vi "ConfigurePigeonMP.vi"(8 "Pigeon Talon":T1, 9 "Pigeon":T6 {"Type" items=["CAN"=352321536, "TalonSRX"=33554432]}, 10 "Right Side":T1, 11 "Left Side":T1) -> (1 "Pigeon":T6 {"Type" items=["CAN"=352321536, "TalonSRX"=33554432]}, 2 "Right Side":T1, 3 "Left Side":T1)   [LabVIEW 2018]
uses:
  <vilib>/Rock Robotics/WPI/ThirdParty/Phoenix-LabVIEW/Pigeon IMU/CTRE_PigeonIMU_DeviceRef.ctl
  <vilib>/Rock Robotics/WPI/ThirdParty/Phoenix-LabVIEW/Pigeon IMU/CTRE_PigeonIMU_ConnectionType.ctl
  <vilib>/Rock Robotics/WPI/MotorControl/WPI_MotorControlDeviceRef.ctl
  <vilib>/Rock Robotics/WPI/MotorControl/WPI_MotorControlType.ctl
  <vilib>/Rock Robotics/SystemInterfaces/DIO/FPGA_DIOPWMChannel.ctl
  <vilib>/Rock Robotics/WPI/PWM/WPI_PWMDeadband.ctl
  <vilib>/Rock Robotics/SystemInterfaces/DIO/FPGA_DIOChannel.ctl
  <vilib>/Rock Robotics/WPI/ThirdParty/Phoenix-LabVIEW/Motor Controller/Controls/CTRE_Phoenix_MotorControl_FeedbackDevice.ctl
  <vilib>/Rock Robotics/WPI/ThirdParty/Phoenix-LabVIEW/Motor Controller/Controls/CTRE_Phoenix_MotorControl_RemoteSourceType.ctl
  <vilib>/Rock Robotics/WPI/ThirdParty/Phoenix-LabVIEW/Motor Controller/Controls/CTRE_Phoenix_MotorControl_SensorTermFeedbackDevice_Enhanced.ctl
  <vilib>/Rock Robotics/WPI/ThirdParty/Phoenix-LabVIEW/Motor Controller/Controls/CTRE_Phoenix_MotorControl_StatusFrameEnhanced.ctl
  <vilib>/Rock Robotics/WPI/ThirdParty/Phoenix-LabVIEW/Motor Controller/Controls/CTRE_Phoenix_MotorControl_NeutralMode.ctl
  <vilib>/Rock Robotics/WPI/ThirdParty/Phoenix-LabVIEW/Motor Controller/Controls/CTRE_Phoenix_MotorControl_ControlMode.ctl
  <vilib>/Rock Robotics/WPI/ThirdParty/Phoenix-LabVIEW/Controls/CTRE_Phoenix_Params.ctl
  <vilib>/Rock Robotics/WPI/ThirdParty/Phoenix-LabVIEW/Motor Controller/Controls/CTRE_Phoenix_MotorControl_ControlFrameEnhanced.ctl
  Constants.vi
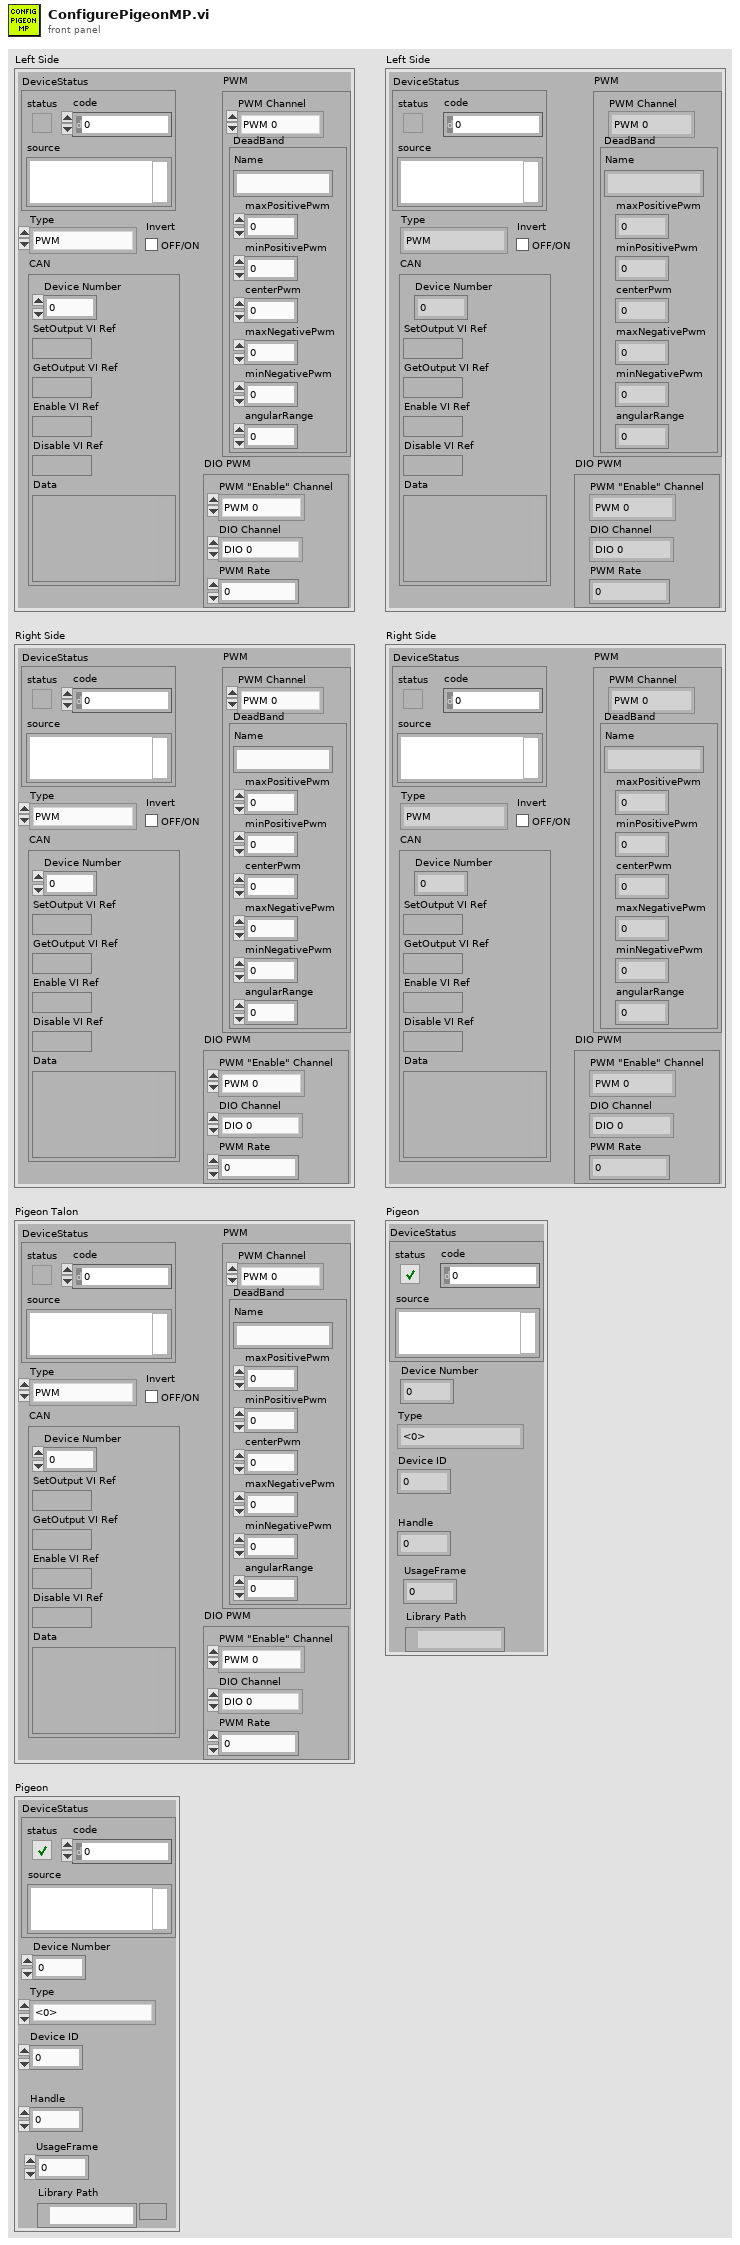
[diagram p1: front panel]
types:
  T1 = typedef "WPI_MotorControlDeviceRef.ctl" = cluster{"DeviceStatus":errorcluster, "Type":T2, "PWM":cluster{"PWM Channel":T3, "DeadBand":T4}, "CAN":cluster{"Device Number":u8, "SetOutput VI Ref":variant, "GetOutput VI Ref":variant, "Enable VI Ref":variant, "Disable VI Ref":variant, "Data":variant}, "Invert":bool, "DIO PWM":cluster{"PWM \"Enable\" Channel":T3, "DIOChannel":T5, "PWM Rate":dbl}}
  T2 = typedef "WPI_MotorControlType.ctl" = enum16{"PWM", "CAN", "DIO PWM"}
  T3 = typedef "FPGA_DIOPWMChannel.ctl" = enum8{"PWM 0", "PWM 1", "PWM 2", "PWM 3", "PWM 4", "PWM 5", "PWM 6", "PWM 7", "PWM 8", "PWM 9", "PWM MXP 0", "PWM MXP 1", "PWM MXP 2", "PWM MXP 3", "PWM MXP 4", "PWM MXP 5", "PWM MXP 6", "PWM MXP 7", "PWM MXP 8", "PWM MXP 9", "Invalid"}
  T4 = typedef "WPI_PWMDeadband.ctl" = cluster{"Name":string, "maxPositivePwm":i32, "minPositivePwm":i32, "centerPwm":i32, "maxNegativePwm":i32, "minNegativePwm":i32, "angularRange":u16}
  T5 = typedef "FPGA_DIOChannel.ctl" = enum8{"DIO 0", "DIO 1", "DIO 2", "DIO 3", "DIO 4", "DIO 5", "DIO 6", "DIO 7", "DIO 8", "DIO 9", "DIO MXP 0", "DIO MXP 1", "DIO MXP 2", "DIO MXP 3", "DIO MXP 4", "DIO MXP 5", "DIO MXP 6", "DIO MXP 7", "DIO MXP 8", "DIO MXP 9", "DIO MXP 10", "DIO MXP 11", "DIO MXP 12", "DIO MXP 13", "DIO MXP 14", "DIO MXP 15", "SPI Port CS1", "SPI Port CS2", "SPI Port CS3", "SPI Port MISO", "SPI Port MOSI", "Invalid"}
  T6 = typedef "CTRE_PigeonIMU_DeviceRef.ctl" = cluster{"DeviceStatus":errorcluster, "Device Number":u8, "Type":T7, "Device ID":u32, "Handle":u64, "UsageFrame":u32, "Library Path":path}
  T7 = typedef "CTRE_PigeonIMU_ConnectionType.ctl" = u32
  T8 = typedef "CTRE_Phoenix_MotorControl_ControlFrameEnhanced.ctl" = u32
  T9 = typedef "CTRE_Phoenix_MotorControl_StatusFrameEnhanced.ctl" = u16
  T10 = typedef "CTRE_Phoenix_Params.ctl" = u16
  T11 = typedef "CTRE_Phoenix_MotorControl_ControlMode.ctl" = u16
  T12 = typedef "CTRE_Phoenix_MotorControl_NeutralMode.ctl" = enum8{"EEPROMSetting", "Override to Coast", "Override to Brake"}
  T13 = typedef "CTRE_Phoenix_MotorControl_FeedbackDevice.ctl" = i8
  T14 = typedef "CTRE_Phoenix_MotorControl_SensorTermFeedbackDevice_Enhanced.ctl" = i8
  T15 = typedef "CTRE_Phoenix_MotorControl_RemoteSourceType.ctl" = enum16{"Off", "Talon SRX Selected Sensor", "Pigeon IMU Yaw", "Pigeon IMU Pitch", "Pigeon IMU Roll", "CANifier Quadrature", "CANifier PWM Input 0", "CANifier PWM Input 1", "CANifier PWM Input 2", "CANifier PWM Input 3", "Gadgeteer Pigeon Yaw", "Gadgeteer Pigeon Pitch", "Gadgeteer Pigeon Roll"}
  T16 = cluster{"kP":dbl, "kI ":dbl, "kD":dbl, "kF":dbl, "I Zone":dbl, "Peak Out":dbl}
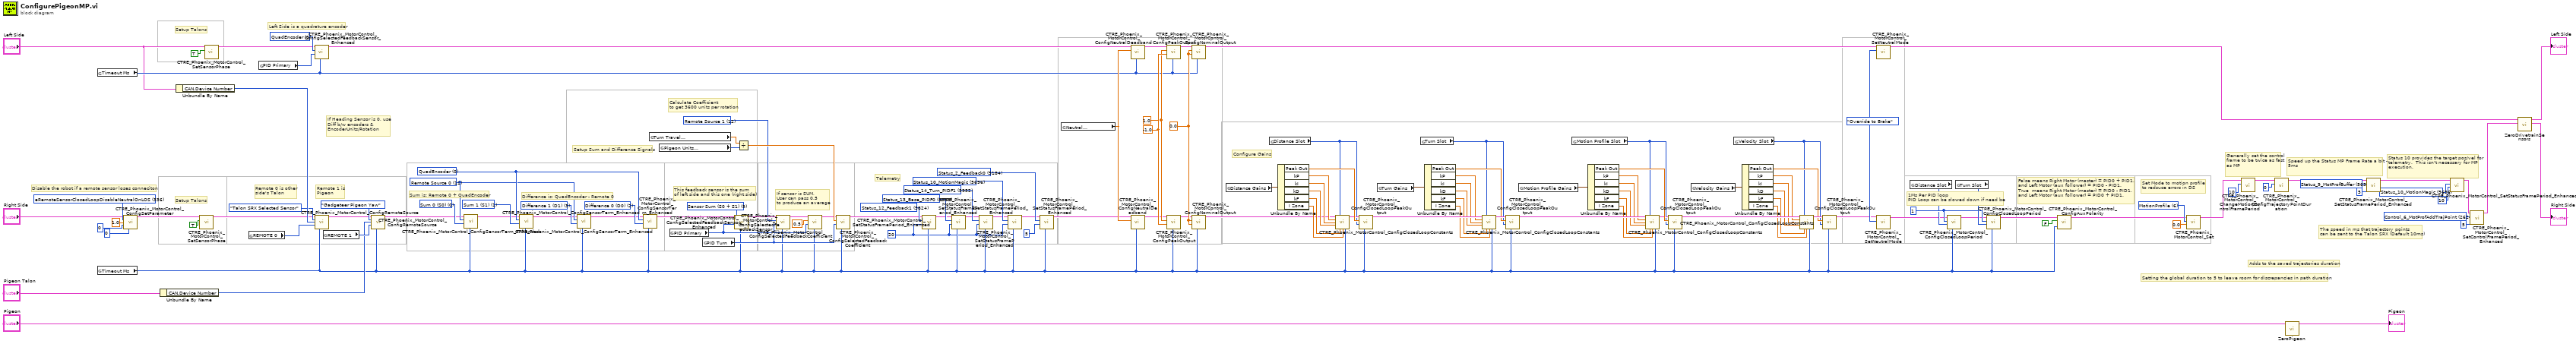
[diagram p0: block diagram]
diagram:
  w8 = T8 262464 items=["Control_3_General"=262272, "Control_4_Advanced"=262336, "Control_5_FeedbackOutputOverride"=262400, "Control_6_MotProfAddTrajPoint"=262464] ("Control Frame")
  w14 = T9 5696 items=["Status_1_General"=5120, "Status_2_Feedback0"=5184, "Status_3_Quadrature"=5248, "Status_4_AinTempVbat"=5312, "Status_6_Misc"=5440, "Status_7_CommStatus"=5504, "Status_8_PulseWidth"=5568, "Status_9_MotProfBuffer"=5632, "Status_10_MotionMagic"=5696, "Status_11_UartGadgeteer"=5760, "Status_12_Feedback1"=5824, "Status_13_Base_PIDF0"=5888, "Status_14_Turn_PIDF1"=5952, "Status_15_FirmwareApiStatus"=6016] ("Status Frame")
  w16 = T9 5632 items=["Status_1_General"=5120, "Status_2_Feedback0"=5184, "Status_3_Quadrature"=5248, "Status_4_AinTempVbat"=5312, "Status_6_Misc"=5440, "Status_7_CommStatus"=5504, "Status_8_PulseWidth"=5568, "Status_9_MotProfBuffer"=5632, "Status_10_MotionMagic"=5696, "Status_11_UartGadgeteer"=5760, "Status_12_Feedback1"=5824, "Status_13_Base_PIDF0"=5888, "Status_14_Turn_PIDF1"=5952, "Status_15_FirmwareApiStatus"=6016] ("Status Frame")
  w21 = T10 336 items=["eOnBoot_BrakeMode"=31, "eQuadFilterEn"=91, "eQuadIdxPolarity"=108, "eClearPositionOnIdx"=100, "eMotionProfileHasUnderrunErr"=119, "eMotionProfileTrajectoryPointDurationMs"=120, "eClearPosOnLimitF"=144, "eClearPosOnLimitR"=145, "eStatusFramePeriod"=300, "eOpenLoopRamp"=301, "eClosedLoopRamp"=302, "eNeutralDeadband"=303, "ePeakPosOutput"=305, "eNominalPosOutput"=306, "ePeakNegOutput"=307, "eNominalNegOutput"=308, "eProfileParamSlot_P"=310, "eProfileParamSlot_I"=311, "eProfileParamSlot_D"=312, "eProfileParamSlot_F"=313, "eProfileParamSlot_IZone"=314, "eProfileParamSlot_AllowableErr"=315, "eProfileParamSlot_MaxIAccum"=316, "eClearPositionOnLimitF"=320, "eClearPositionOnLimitR"=321, "eClearPositionOnQuadIdx"=322, "eSampleVelocityPeriod"=325, "eSampleVelocityWindow"=326, "eFeedbackSensorType"=330, "eSelectedSensorPosition"=331, "eFeedbackNotContinuous"=332, "eRemoteSensorSource"=333, "eRemoteSensorDeviceID"=334, "eSensorTerm"=335, "eRemoteSensorClosedLoopDisableNeutralOnLOS"=336, "eForwardSoftLimitThreshold"=340, "eReverseSoftLimitThreshold"=341, "eForwardSoftLimitEnable"=342, "eReverseSoftLimitEnable"=343, "eNominalBatteryVoltage"=350, "eBatterVoltageFilterSize"=351, "eContinuousCurrentLimitAmps"=360, "eContinuousCurrentLimitMs"=361, "ePeakCurrentLimitAmps"=362, "eClosedLoopIAccum"=370, "eCustomParam"=380, "eStickyFaults"=390, "eAnalogPosition"=400, "eQuadraturePosition"=401, "ePulseWidthPosition"=402, "eMotMag_Accel"=410, "eMotMag_VelCruise"=411, "eLimitSwitchSource"=421, "eLimitSwitchNormClosedAndDis"=422, "eLimitSwitchDisabledNeutralOnLOS"=423, "eLimitSwitchRemoteDevID"=424] ("Parameter")
  w33 = T11 6 items=["PercentOutput"=0, "Position"=1, "Velocity"=2, "Current"=3, "Follower"=5, "MotionProfile"=6, "MotionMagic"=7, "MotionProfileArc"=10, "Disabled"=15] ("Control Mode")
  w136 = 1 ("loopTimeMs")
  w132 = CTRE_Phoenix_MotorControl_NeutralMode."Override to Brake" ("Motor Control Neutral Mode")
  w93 = 0.0 ("Forward Nominal Percent Output")
  w90 = -1.0 ("Reverse Peak Percent Output")
  w89 = 1.0 ("Forward Peak Percent Output")
  w30 = 20 ("periodMs")
  w82 = T9 5184 items=["Status_1_General"=5120, "Status_2_Feedback0"=5184, "Status_3_Quadrature"=5248, "Status_4_AinTempVbat"=5312, "Status_6_Misc"=5440, "Status_7_CommStatus"=5504, "Status_8_PulseWidth"=5568, "Status_9_MotProfBuffer"=5632, "Status_10_MotionMagic"=5696, "Status_11_UartGadgeteer"=5760, "Status_12_Feedback1"=5824, "Status_13_Base_PIDF0"=5888, "Status_14_Turn_PIDF1"=5952, "Status_15_FirmwareApiStatus"=6016] ("Status Frame")
  w81 = T9 5696 items=["Status_1_General"=5120, "Status_2_Feedback0"=5184, "Status_3_Quadrature"=5248, "Status_4_AinTempVbat"=5312, "Status_6_Misc"=5440, "Status_7_CommStatus"=5504, "Status_8_PulseWidth"=5568, "Status_9_MotProfBuffer"=5632, "Status_10_MotionMagic"=5696, "Status_11_UartGadgeteer"=5760, "Status_12_Feedback1"=5824, "Status_13_Base_PIDF0"=5888, "Status_14_Turn_PIDF1"=5952, "Status_15_FirmwareApiStatus"=6016] ("Status Frame")
  w80 = T9 5952 items=["Status_1_General"=5120, "Status_2_Feedback0"=5184, "Status_3_Quadrature"=5248, "Status_4_AinTempVbat"=5312, "Status_6_Misc"=5440, "Status_7_CommStatus"=5504, "Status_8_PulseWidth"=5568, "Status_9_MotProfBuffer"=5632, "Status_10_MotionMagic"=5696, "Status_11_UartGadgeteer"=5760, "Status_12_Feedback1"=5824, "Status_13_Base_PIDF0"=5888, "Status_14_Turn_PIDF1"=5952, "Status_15_FirmwareApiStatus"=6016] ("Status Frame")
  w79 = T9 5888 items=["Status_1_General"=5120, "Status_2_Feedback0"=5184, "Status_3_Quadrature"=5248, "Status_4_AinTempVbat"=5312, "Status_6_Misc"=5440, "Status_7_CommStatus"=5504, "Status_8_PulseWidth"=5568, "Status_9_MotProfBuffer"=5632, "Status_10_MotionMagic"=5696, "Status_11_UartGadgeteer"=5760, "Status_12_Feedback1"=5824, "Status_13_Base_PIDF0"=5888, "Status_14_Turn_PIDF1"=5952, "Status_15_FirmwareApiStatus"=6016] ("Status Frame")
  w78 = T9 5824 items=["Status_1_General"=5120, "Status_2_Feedback0"=5184, "Status_3_Quadrature"=5248, "Status_4_AinTempVbat"=5312, "Status_6_Misc"=5440, "Status_7_CommStatus"=5504, "Status_8_PulseWidth"=5568, "Status_9_MotProfBuffer"=5632, "Status_10_MotionMagic"=5696, "Status_11_UartGadgeteer"=5760, "Status_12_Feedback1"=5824, "Status_13_Base_PIDF0"=5888, "Status_14_Turn_PIDF1"=5952, "Status_15_FirmwareApiStatus"=6016] ("Status Frame")
  w28 = T13 12 items=["None"=-1, "QuadEncoder"=0, "Analog"=2, "Tachometer"=4, "Pulse Width Encoded Position"=8, "Sensor Sum (S0 + S1)"=9, "Sensor Difference (D0 - D1)"=10, "Remote Source 0"=11, "Remote Source 1"=12, "Software Emulated"=15] ("Feedback Device")
  w65 = T13 9 items=["None"=-1, "QuadEncoder"=0, "Analog"=2, "Tachometer"=4, "Pulse Width Encoded Position"=8, "Sensor Sum (S0 + S1)"=9, "Sensor Difference (D0 - D1)"=10, "Remote Source 0"=11, "Remote Source 1"=12, "Software Emulated"=15] ("Feedback Device")
  w63 = u16 2 items=["Sum 0 (S0)", "Sum 1 (S1)", "Difference 0 (D0)", "Difference 1 (D1)"] ("Sensor Term")
  w62 = u16 3 items=["Sum 0 (S0)", "Sum 1 (S1)", "Difference 0 (D0)", "Difference 1 (D1)"] ("Sensor Term")
  w57 = u16 1 items=["Sum 0 (S0)", "Sum 1 (S1)", "Difference 0 (D0)", "Difference 1 (D1)"] ("Sensor Term")
  w61 = T14 0 items=["None"=-1, "QuadEncoder"=0, "Analog"=2, "Tachometer"=4, "Pulse Width Encoded Position"=8, "Remote Source 0"=11, "Remote Source 1"=12, "Software Emulated"=15] ("Feedback Device")
  w55 = u16 0 items=["Sum 0 (S0)", "Sum 1 (S1)", "Difference 0 (D0)", "Difference 1 (D1)"] ("Sensor Term")
  w60 = T14 11 items=["None"=-1, "QuadEncoder"=0, "Analog"=2, "Tachometer"=4, "Pulse Width Encoded Position"=8, "Remote Source 0"=11, "Remote Source 1"=12, "Software Emulated"=15] ("Feedback Device")
  w44 = T13 0 items=["None"=-1, "QuadEncoder"=0, "Analog"=2, "Tachometer"=4, "Pulse Width Encoded Position"=8, "Sensor Sum (S0 + S1)"=9, "Sensor Difference (D0 - D1)"=10, "Remote Source 0"=11, "Remote Source 1"=12, "Software Emulated"=15] ("Feedback Device")
  # "Setting the global duration to 5 to leave room for discrepancies in path duration"
  # "Adds to the saved trajectories duration"
  # "The speed in ms that trajectory points\ncan be sent to the Talon SRX (Default 10ms)"
  # "Generally set the control frame to be twice as fast as MP"
  # "Status 10 provides the target pos/vel for telemetry.  This isn't necessary for MP execution."
  # "Speed up the Status MP Frame Rate a bit - 5ms"
  # "Disable the robot if a remote sensor loses conneciton"
  # "Set Mode to motion profile\nto redsuce errors in DS"
  # "False means Right Motor (master) = PID0 + PID1, \nand Left Motor (aux follower) = PID0 - PID1.\nTrue  means Right Motor (master) = PID0 - PID1, \nand Left Motor (aux follower) = PID0 + PID1."
  # "1Ms Per PID loop\nPID Loop can be slowed down if need be"
  # "Configure Gains"
  # "Setup Talons"
  # "Telemetry"
  # "If sensor is SUM,\nUser can pass 0.5\nto produce an average"
  # "Calculate Coefficient\nto get 3600 units per rotation"
  # "If Heading Sensor is 0, use \nDiff b/w encoders &\nEncoderUnits/Rotation"
  # "This feedback sensor is the sum\nof left side and this one (right side)"
  # "Difference is: QuadEncoder - Remote 0"
  # "Sum is: Remote 0 + QuadEncoder"
  # "Setup Sum and Difference Signals"
  # "Remote 1 is\nPigeon"
  # "Remote 0 is other\nside's Talon"
  # "Left Side is a quadrature encoder"
  # "Setup Talons"
  n1 = global read "Constants.vi" "Timeout Ms"() -> (w27:i32)
  n2 = global read "Constants.vi" "Timeout Ms"() -> (w39:i32)
  n3 = call <vilib>:"CTRE_Phoenix_MotorControl_ConfigSetParameter.vi"("PhoenixMotorControlDevRef"="Right Side", "Parameter"=w21, "value"=1.0, "subValue"=u8 0, "ordinal"=0) -> ("PhoenixMotorControlDevRef"=w2:T1)  [unwired: 9 in, 1 out]
  n4 = Unbundle By Name("Pigeon Talon") -> ("CAN.Device Number"=w52:u8)
  n5 = Unbundle By Name("Left Side") -> ("CAN.Device Number"=w47:u8)
  n6 = call <vilib>:"CTRE_Phoenix_MotorControl_SetSensorPhase.vi"("PhaseSensor"=TRUE, "PhoenixMotorControlDevRef"=w2) -> ("PhoenixMotorControlDevRef"=w45:T1)  [unwired: 8 in, 1 out]
  n7 = call <vilib>:"CTRE_Phoenix_MotorControl_SetSensorPhase.vi"("PhaseSensor"=TRUE, "PhoenixMotorControlDevRef"="Left Side") -> ("PhoenixMotorControlDevRef"=w43:T1)  [unwired: 8 in, 1 out]
  n8 = global read "Constants.vi" "REMOTE 0"() -> (w48:i32)
  n9 = global read "Constants.vi" "PID Primary"() -> (w139:i32)
  n10 = call <vilib>:"CTRE_Phoenix_MotorControl_ConfigSelectedFeedbackSensor_Enhanced.vi"("timeoutMs"=w27, "pidLoopIdx"=w139, "Feedback Device"=w44, "PhoenixMotorControlDevRef"=w43) -> ("PhoenixMotorControlDevRef"=w86:T1)  [unwired: 6 in, 1 out]
  n11 = call <vilib>:"CTRE_Phoenix_MotorControl_ConfigRemoteSource.vi"("PhoenixMotorControlDevRef"=w45, "Remote Device Type"=CTRE_Phoenix_MotorControl_RemoteSourceType."Talon SRX Selected Sensor", "Remote Device ID"=w47, "Source Index (0/1)"=w48, "timeoutMs"=w39) -> ("PhoenixMotorControlDevRef"=w49:T1)  [unwired: 9 in, 1 out]
  n12 = global read "Constants.vi" "REMOTE 1"() -> (w53:i32)
  n13 = call <vilib>:"CTRE_Phoenix_MotorControl_ConfigRemoteSource.vi"("PhoenixMotorControlDevRef"=w49, "Remote Device Type"=CTRE_Phoenix_MotorControl_RemoteSourceType."Gadgeteer Pigeon Yaw", "Remote Device ID"=w52, "Source Index (0/1)"=w53, "timeoutMs"=w39) -> ("PhoenixMotorControlDevRef"=w54:T1)  [unwired: 9 in, 1 out]
  n14 = call <vilib>:"CTRE_Phoenix_MotorControl_ConfigSensorTerm_Enhanced.vi"("timeoutMs"=w39, "Sensor Term"=w55, "Feedback Device"=w60, "PhoenixMotorControlDevRef"=w54) -> ("PhoenixMotorControlDevRef"=w56:T1)  [unwired: 6 in, 1 out]
  n15 = call <vilib>:"CTRE_Phoenix_MotorControl_ConfigSensorTerm_Enhanced.vi"("timeoutMs"=w39, "Sensor Term"=w57, "Feedback Device"=w61, "PhoenixMotorControlDevRef"=w56) -> ("PhoenixMotorControlDevRef"=w59:T1)  [unwired: 6 in, 1 out]
  n16 = call <vilib>:"CTRE_Phoenix_MotorControl_ConfigSensorTerm_Enhanced.vi"("timeoutMs"=w39, "Sensor Term"=w62, "Feedback Device"=w60, "PhoenixMotorControlDevRef"=w59) -> ("PhoenixMotorControlDevRef"=w58:T1)  [unwired: 6 in, 1 out]
  n17 = call <vilib>:"CTRE_Phoenix_MotorControl_ConfigSensorTerm_Enhanced.vi"("timeoutMs"=w39, "Sensor Term"=w63, "Feedback Device"=w61, "PhoenixMotorControlDevRef"=w58) -> ("PhoenixMotorControlDevRef"=w64:T1)  [unwired: 6 in, 1 out]
  n18 = global read "Constants.vi" "Turn Travel\nUnits Per Rotation"() -> (w71:dbl)
  n19 = global read "Constants.vi" "Pigeon Units\nPer Rotatoin"() -> (w29:i32)
  n20 = global read "Constants.vi" "PID Primary"() -> (w138:i32)
  n21 = global read "Constants.vi" "PID Turn"() -> (w70:i32)
  n22 = call <vilib>:"CTRE_Phoenix_MotorControl_ConfigSelectedFeedbackSensor_Enhanced.vi"("timeoutMs"=w39, "pidLoopIdx"=w138, "Feedback Device"=w65, "PhoenixMotorControlDevRef"=w64) -> ("PhoenixMotorControlDevRef"=w66:T1)  [unwired: 6 in, 1 out]
  n23 = Divide(x=w71, y=w29) -> (x/y=w72:dbl)
  n24 = call <vilib>:"CTRE_Phoenix_MotorControl_ConfigSelectedFeedbackSensor_Enhanced.vi"("timeoutMs"=w39, "pidLoopIdx"=w70, "Feedback Device"=w28, "PhoenixMotorControlDevRef"=w66) -> ("PhoenixMotorControlDevRef"=w67:T1)  [unwired: 6 in, 1 out]
  n25 = call <vilib>:"CTRE_Phoenix_MotorControl_ConfigSelectedFeedbackCoefficient.vi"("timoutMs"=w39, "pidIdx"=w138, "coefficient"=0.5, "PhoenixMotorControlDevRef"=w67) -> ("PhoenixMotorControlDevRef"=w69:T1)  [unwired: 6 in, 1 out]
  n26 = call <vilib>:"CTRE_Phoenix_MotorControl_ConfigSelectedFeedbackCoefficient.vi"("timoutMs"=w39, "pidIdx"=w70, "coefficient"=w72, "PhoenixMotorControlDevRef"=w69) -> ("PhoenixMotorControlDevRef"=w73:T1)  [unwired: 6 in, 1 out]
  n27 = call <vilib>:"CTRE_Phoenix_MotorControl_SetStatusFramePeriod_Enhanced.vi"("timeoutMs"=w39, "periodMs"=w30, "Status Frame"=w78, "PhoenixMotorControlDevRef"=w73) -> ("PhoenixMotorControlDevRef"=w74:T1)  [unwired: 6 in, 1 out]
  n28 = call <vilib>:"CTRE_Phoenix_MotorControl_SetStatusFramePeriod_Enhanced.vi"("timeoutMs"=w39, "periodMs"=w30, "Status Frame"=w79, "PhoenixMotorControlDevRef"=w74) -> ("PhoenixMotorControlDevRef"=w75:T1)  [unwired: 6 in, 1 out]
  n29 = call <vilib>:"CTRE_Phoenix_MotorControl_SetStatusFramePeriod_Enhanced.vi"("timeoutMs"=w39, "periodMs"=w30, "Status Frame"=w80, "PhoenixMotorControlDevRef"=w75) -> ("PhoenixMotorControlDevRef"=w76:T1)  [unwired: 6 in, 1 out]
  n30 = call <vilib>:"CTRE_Phoenix_MotorControl_SetStatusFramePeriod_Enhanced.vi"("timeoutMs"=w39, "periodMs"=w30, "Status Frame"=w81, "PhoenixMotorControlDevRef"=w76) -> ("PhoenixMotorControlDevRef"=w77:T1)  [unwired: 6 in, 1 out]
  n31 = call <vilib>:"CTRE_Phoenix_MotorControl_SetStatusFramePeriod_Enhanced.vi"("timeoutMs"=w39, "periodMs"=5, "Status Frame"=w82, "PhoenixMotorControlDevRef"=w77) -> ("PhoenixMotorControlDevRef"=w84:T1)  [unwired: 6 in, 1 out]
  n32 = global read "Constants.vi" "Neutral\nDeadband"() -> (w87:dbl)
  n33 = call <vilib>:"CTRE_Phoenix_MotorControl_ConfigNeutralDeadband.vi"("timeoutMs"=w27, "Percent Deadband"=w87, "PhoenixMotorControlDevRef"=w86) -> ("PhoenixMotorControlDevRef"=w88:T1)  [unwired: 7 in, 1 out]
  n34 = call <vilib>:"CTRE_Phoenix_MotorControl_ConfigNeutralDeadband.vi"("timeoutMs"=w39, "Percent Deadband"=w87, "PhoenixMotorControlDevRef"=w84) -> ("PhoenixMotorControlDevRef"=w85:T1)  [unwired: 7 in, 1 out]
  n35 = call <vilib>:"CTRE_Phoenix_MotorControl_ConfigPeakOutput.vi"("timeoutMs"=w27, "Reverse Peak Percent Output"=w90, "Forward Peak Percent Output"=w89, "PhoenixMotorControlDevRef"=w88) -> ("PhoenixMotorControlDevRef"=w92:T1)  [unwired: 6 in, 1 out]
  n36 = call <vilib>:"CTRE_Phoenix_MotorControl_ConfigPeakOutput.vi"("timeoutMs"=w39, "Reverse Peak Percent Output"=w90, "Forward Peak Percent Output"=w89, "PhoenixMotorControlDevRef"=w85) -> ("PhoenixMotorControlDevRef"=w91:T1)  [unwired: 6 in, 1 out]
  n37 = call <vilib>:"CTRE_Phoenix_MotorControl_ConfigNominalOutput.vi"("timeoutMs"=w27, "Reverse Nominal Percent Output"=w93, "Forward Nominal Percent Output"=w93, "PhoenixMotorControlDevRef"=w92) -> ("PhoenixMotorControlDevRef"=w131:T1)  [unwired: 6 in, 1 out]
  n38 = call <vilib>:"CTRE_Phoenix_MotorControl_ConfigNominalOutput.vi"("timeoutMs"=w39, "Reverse Nominal Percent Output"=w93, "Forward Nominal Percent Output"=w93, "PhoenixMotorControlDevRef"=w91) -> ("PhoenixMotorControlDevRef"=w94:T1)  [unwired: 6 in, 1 out]
  n39 = global read "Constants.vi" "Distance Gains"() -> (w95:T16)
  n40 = global read "Constants.vi" "Distance Slot"() -> (w36:i32)
  n41 = Unbundle By Name(w95) -> ("Peak Out"=w102:dbl, "kP"=w96:dbl, "kI"=w97:dbl, "kD"=w98:dbl, "kF"=w99:dbl, "I Zone"=w100:dbl)
  n42 = call <vilib>:"CTRE_Phoenix_MotorControl_ConfigClosedLoopConstants.vi"("PhoenixMotorControlDevRef"=w94, "slotIdx"=w36, "P"=w96, "I"=w97, "D"=w98, "F"=w99, "I Zone"=w100, "timeoutMs"=w39) -> ("PhoenixMotorControlDevRef"=w101:T1)  [unwired: 6 in, 1 out]
  n43 = call <vilib>:"CTRE_Phoenix_MotorControl_ConfigClosedLoopPeakOutput.vi"("timoutMs"=w39, "slotIdx"=w36, "peakOutput"=w102, "PhoenixMotorControlDevRef"=w101) -> ("PhoenixMotorControlDevRef"=w127:T1)  [unwired: 6 in, 1 out]
  n44 = global read "Constants.vi" "Turn Gains"() -> (w110:T16)
  n45 = global read "Constants.vi" "Turn Slot"() -> (w35:i32)
  n46 = Unbundle By Name(w110) -> ("Peak Out"=w103:dbl, "kP"=w109:dbl, "kI"=w108:dbl, "kD"=w107:dbl, "kF"=w106:dbl, "I Zone"=w105:dbl)
  n47 = call <vilib>:"CTRE_Phoenix_MotorControl_ConfigClosedLoopConstants.vi"("PhoenixMotorControlDevRef"=w127, "slotIdx"=w35, "P"=w109, "I"=w108, "D"=w107, "F"=w106, "I Zone"=w105, "timeoutMs"=w39) -> ("PhoenixMotorControlDevRef"=w104:T1)  [unwired: 6 in, 1 out]
  n48 = call <vilib>:"CTRE_Phoenix_MotorControl_ConfigClosedLoopPeakOutput.vi"("timoutMs"=w39, "slotIdx"=w35, "peakOutput"=w103, "PhoenixMotorControlDevRef"=w104) -> ("PhoenixMotorControlDevRef"=w128:T1)  [unwired: 6 in, 1 out]
  n49 = global read "Constants.vi" "Motion Profile Gains"() -> (w111:T16)
  n50 = global read "Constants.vi" "Motion Profile Slot"() -> (w37:i32)
  n51 = Unbundle By Name(w111) -> ("Peak Out"=w118:dbl, "kP"=w112:dbl, "kI"=w113:dbl, "kD"=w114:dbl, "kF"=w115:dbl, "I Zone"=w116:dbl)
  n52 = call <vilib>:"CTRE_Phoenix_MotorControl_ConfigClosedLoopConstants.vi"("PhoenixMotorControlDevRef"=w128, "slotIdx"=w37, "P"=w112, "I"=w113, "D"=w114, "F"=w115, "I Zone"=w116, "timeoutMs"=w39) -> ("PhoenixMotorControlDevRef"=w117:T1)  [unwired: 6 in, 1 out]
  n53 = call <vilib>:"CTRE_Phoenix_MotorControl_ConfigClosedLoopPeakOutput.vi"("timoutMs"=w39, "slotIdx"=w37, "peakOutput"=w118, "PhoenixMotorControlDevRef"=w117) -> ("PhoenixMotorControlDevRef"=w129:T1)  [unwired: 6 in, 1 out]
  n54 = global read "Constants.vi" "Velocity Gains"() -> (w126:T16)
  n55 = global read "Constants.vi" "Velocity Slot"() -> (w34:i32)
  n56 = Unbundle By Name(w126) -> ("Peak Out"=w119:dbl, "kP"=w125:dbl, "kI"=w124:dbl, "kD"=w123:dbl, "kF"=w122:dbl, "I Zone"=w121:dbl)
  n57 = call <vilib>:"CTRE_Phoenix_MotorControl_ConfigClosedLoopConstants.vi"("PhoenixMotorControlDevRef"=w129, "slotIdx"=w34, "P"=w125, "I"=w124, "D"=w123, "F"=w122, "I Zone"=w121, "timeoutMs"=w39) -> ("PhoenixMotorControlDevRef"=w120:T1)  [unwired: 6 in, 1 out]
  n58 = call <vilib>:"CTRE_Phoenix_MotorControl_ConfigClosedLoopPeakOutput.vi"("timoutMs"=w39, "slotIdx"=w34, "peakOutput"=w119, "PhoenixMotorControlDevRef"=w120) -> ("PhoenixMotorControlDevRef"=w130:T1)  [unwired: 6 in, 1 out]
  n59 = call <vilib>:"CTRE_Phoenix_MotorControl_SetNeutralMode.vi"("Motor Control Neutral Mode"=w132, "PhoenixMotorControlDevRef"=w131) -> ("PhoenixMotorControlDevRef"=w24:T1)  [unwired: 8 in, 1 out]
  n60 = call <vilib>:"CTRE_Phoenix_MotorControl_SetNeutralMode.vi"("Motor Control Neutral Mode"=w132, "PhoenixMotorControlDevRef"=w130) -> ("PhoenixMotorControlDevRef"=w133:T1)  [unwired: 8 in, 1 out]
  n61 = global read "Constants.vi" "Distance Slot"() -> (w134:i32)
  n62 = call <vilib>:"CTRE_Phoenix_MotorControl_ConfigClosedLoopPeriod.vi"("timoutMs"=w39, "slotIdx"=w134, "loopTimeMs"=w136, "PhoenixMotorControlDevRef"=w133) -> ("PhoenixMotorControlDevRef"=w135:T1)  [unwired: 6 in, 1 out]
  n63 = global read "Constants.vi" "Turn Slot"() -> (w137:i32)
  n64 = call <vilib>:"CTRE_Phoenix_MotorControl_ConfigClosedLoopPeriod.vi"("timoutMs"=w39, "slotIdx"=w137, "loopTimeMs"=w136, "PhoenixMotorControlDevRef"=w135) -> ("PhoenixMotorControlDevRef"=w40:T1)  [unwired: 6 in, 1 out]
  n65 = call <vilib>:"CTRE_Phoenix_MotorControl_ConfigAuxPolarity.vi"("timeoutMs"=w39, "Invert"=FALSE, "PhoenixMotorControlDevRef"=w40) -> ("PhoenixMotorControlDevRef"=w31:T1)  [unwired: 7 in, 1 out]
  n66 = call <vilib>:"CTRE_Phoenix_MotorControl_Set.vi"("Output"=0.0, "Control Mode"=w33, "PhoenixMotorControlDevRef"=w31) -> ("PhoenixMotorControlDevRef"=w5:T1)  [unwired: 7 in, 1 out]
  n67 = call <vilib>:"CTRE_Phoenix_MotorControl_ChangeMotionControlFramePeriod.vi"("periodMs"=10, "PhoenixMotorControlDevRef"=w5) -> ("PhoenixMotorControlDevRef"=w11:T1)  [unwired: 8 in, 1 out]
  n68 = call <vilib>:"CTRE_Phoenix_MotorControl_ConfigTrajectoryPointDuration.vi"("durationMs"=0, "PhoenixMotorControlDevRef"=w11) -> ("PhoenixMotorControlDevRef"=w10:T1)  [unwired: 8 in, 1 out]
  n69 = call "ZeroPigeon.vi"("Pigeon"="Pigeon") -> ("Pigeon"=→"Pigeon":T6)  [unwired: 8 in]
  n70 = call <vilib>:"CTRE_Phoenix_MotorControl_SetStatusFramePeriod_Enhanced.vi"("periodMs"=5, "Status Frame"=w16, "PhoenixMotorControlDevRef"=w10) -> ("PhoenixMotorControlDevRef"=w12:T1)  [unwired: 7 in, 1 out]
  n71 = call <vilib>:"CTRE_Phoenix_MotorControl_SetStatusFramePeriod_Enhanced.vi"("periodMs"=10, "Status Frame"=w14, "PhoenixMotorControlDevRef"=w12) -> ("PhoenixMotorControlDevRef"=w7:T1)  [unwired: 7 in, 1 out]
  n72 = call <vilib>:"CTRE_Phoenix_MotorControl_SetControlFramePeriod_Enhanced.vi"("periodMs"=5, "Control Frame"=w8, "MotorControl Device Ref"=w7) -> ("PhoenixMotorControlDevRef"=w4:T1)  [unwired: 7 in, 1 out]
  n73 = call "ZeroDrivetrainSensors.vi"("Talon 2"=w4, "Talon 1"=w24) -> ("Talon 2"=→"Right Side":T1, "Talon 1"=→"Left Side":T1)  [unwired: 8 in]
